vi "XIPIN_3GPP_LTE_Channel_Estimator_1_1.vi"   [LabVIEW 2017]
doc: "The 3GPP LTE Channel Estimator v1.1 core implements channel estimation functionality for uplink LTE eNodeB applications based on the 3GPP TS 36.211 specification.\n------------------------------------\n<b>Need License</b> : Yes\n<b>Interface</b> : AXI4-Stream"
uses:
  <vilib>/rvi/XilinxIP/XIPIN_XNode/niFpgaXIPIN.xnode
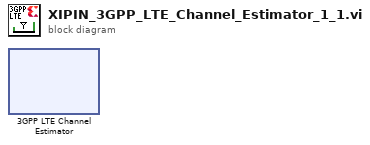
[diagram p0: block diagram]
diagram:
  n1 = xnode ("3GPP LTE Channel Estimator")() -> ()
